vi "Stimulus.Create.vi"(8 "error in (no error)":errorcluster, 11 "State Variables":T1={"NIVS.BaseLogPath"=path "", "NIVS.SystemDefinitionFile"=path "", "NIVS.Events"={"SequenceEvent"=refnum, "SystemChangeEvent"=refnum, "WorkspaceEvent"=refnum}, "NIVS.SequenceState"=enum."Idle", "NIVS.GatewayIPAddress"="", "NIVS.DataLogSpecRef"=refnum, "NIVS.DataLogManagerRef"=refnum, "NIVS.LogSessionGUID"="", "NIVS.WorkspaceManager"=refnum, "NIVS.Deployed"=FALSE, "NIVS.ProfileRef"=refnum, "NIVS.ProfileCallback"=refnum, "NIVS.SystemStateRefs"={"CustDatRef"=refnum, "EvtRef"=refnum, "Target State User Event"=refnum}, "UI.Abort"=refnum, "UI.Pause"=refnum, "UI.EnableLogging"=refnum, "UI.Start"=refnum, "UI.LogChannels"=refnum, "UI.StartIteration"=refnum, "UI.StartStep"=refnum, "UI.Sequence"=refnum, "UI.PreviewMode"=refnum, "UI.Graph"=refnum, "UI.BaseFileName"=refnum, "UI.Profiles"=refnum, "UI.CurrentStep"=refnum, "UI.CurrentIteration"=refnum, "UI.TotalIterations"=refnum, "Sequence.AbortChannel"="", "Sequence.StepInfoChannel"="", "Sequence.Iterations"=0, "Sequence.IterationInfoChannel"="", "Sequence.#ofColumns"=0, "Events.State"=refnum, "Events.Test Result"=refnum, "Events.Progress"=refnum, "INI.Settings"={"Build Location"=path "C:/Simple Sequence Editor/SequenceRepo", "LoggingLocation"=path ""}, "UI.Skip"=refnum, "Sequence.SkipChannel"="", "Restart.Path"=path "", "UI.Duration"=refnum, "Sequence.DurationChannel"=""}) -> (0 "error out":errorcluster, 3 "State Variables":T1={"NIVS.BaseLogPath"=path "", "NIVS.SystemDefinitionFile"=path "", "NIVS.Events"={"SequenceEvent"=refnum, "SystemChangeEvent"=refnum, "WorkspaceEvent"=refnum}, "NIVS.SequenceState"=enum."Idle", "NIVS.GatewayIPAddress"="", "NIVS.DataLogSpecRef"=refnum, "NIVS.DataLogManagerRef"=refnum, "NIVS.LogSessionGUID"="", "NIVS.WorkspaceManager"=refnum, "NIVS.Deployed"=FALSE, "NIVS.ProfileRef"=refnum, "NIVS.ProfileCallback"=refnum, "NIVS.SystemStateRefs"={"CustDatRef"=refnum, "EvtRef"=refnum, "Target State User Event"=refnum}, "UI.Abort"=refnum, "UI.Pause"=refnum, "UI.EnableLogging"=refnum, "UI.Start"=refnum, "UI.LogChannels"=refnum, "UI.StartIteration"=refnum, "UI.StartStep"=refnum, "UI.Sequence"=refnum, "UI.PreviewMode"=refnum, "UI.Graph"=refnum, "UI.BaseFileName"=refnum, "UI.Profiles"=refnum, "UI.CurrentStep"=refnum, "UI.CurrentIteration"=refnum, "UI.TotalIterations"=refnum, "Sequence.AbortChannel"="", "Sequence.StepInfoChannel"="", "Sequence.Iterations"=0, "Sequence.IterationInfoChannel"="", "Sequence.#ofColumns"=0, "Events.State"=refnum, "Events.Test Result"=refnum, "Events.Progress"=refnum, "INI.Settings"={"Build Location"=path "C:/Simple Sequence Editor/SequenceRepo", "LoggingLocation"=path ""}, "UI.Skip"=refnum, "Sequence.SkipChannel"="", "Restart.Path"=path "", "UI.Duration"=refnum, "Sequence.DurationChannel"=""})   [LabVIEW 2015, in "Simple Sequence Tools - Execution.lvlib"]
uses:
  Simple Sequence Tools - Execution.lvlib
  Types/Main.StateVariables.ctl
  Types/Execute.UserEventRefs.ctl
  <vilib>/NI Veristand/Execution/Workspace/SystemStateRegEventRef.ctl
  <vilib>/NI Veristand/Execution/Workspace/Target State Info.ctl
  <vilib>/NI Veristand/Execution/Workspace/Target State.ctl
  Types/Execution.SequenceState.ctl
  <vilib>/NI Veristand/Execution/DataLogging/DataLoggingSpecification Ref.ctl
  NationalInstruments.VeriStand.ClientAPI
  <vilib>/NI Veristand/Execution/DataLogging/IDataLogging Ref.ctl
  <vilib>/NI Veristand/Execution/Workspace/WorkspaceAPI.ctl
  NationalInstruments.VeriStand.RealTimeSequenceDefinitionApi
  <vilib>/NI Veristand/Execution/Workspace/SystemStateEventRef.ctl
  Shared/Types/INI.Settings
  Types/Restart.Settings
  <vilib>/NI Veristand/Execution/DataLogging/TDMS Channel Group.ctl
  <vilib>/NI Veristand/Execution/DataLogging/TDMS Property.ctl
  <vilib>/NI Veristand/Execution/DataLogging/TDMS Channel.ctl
  <vilib>/NI Veristand/Execution/DataLogging/Time Channel Options.ctl
  Types/Log.SelectedChannels.ctl
  NationalInstruments.VeriStand
  NationalInstruments.VeriStand.DataTypes
  <vilib>/NI Veristand/Execution/DataLogging/File Conflict Operation.ctl
  Shared/SubVIs/Main.Constants.vi
  <vilib>/NI Veristand/Execution/DataLogging/New Data Logging Specification (TDMS).vi
  <vilib>/NI Veristand/Execution/DataLogging/Set Data Logging Rate (Target Rate).vi
  <vilib>/NI Veristand/Execution/DataLogging/Set Start Trigger (Start Immediately).vi
  <vilib>/NI Veristand/Execution/Workspace/NI_VS Workspace ExecutionAPI.lvlib
  Shared/Simple Sequence Tools - Shared.lvlib
  <vilib>/NI Veristand/Execution/DataLogging/NI_VS Data Logging API.lvlib
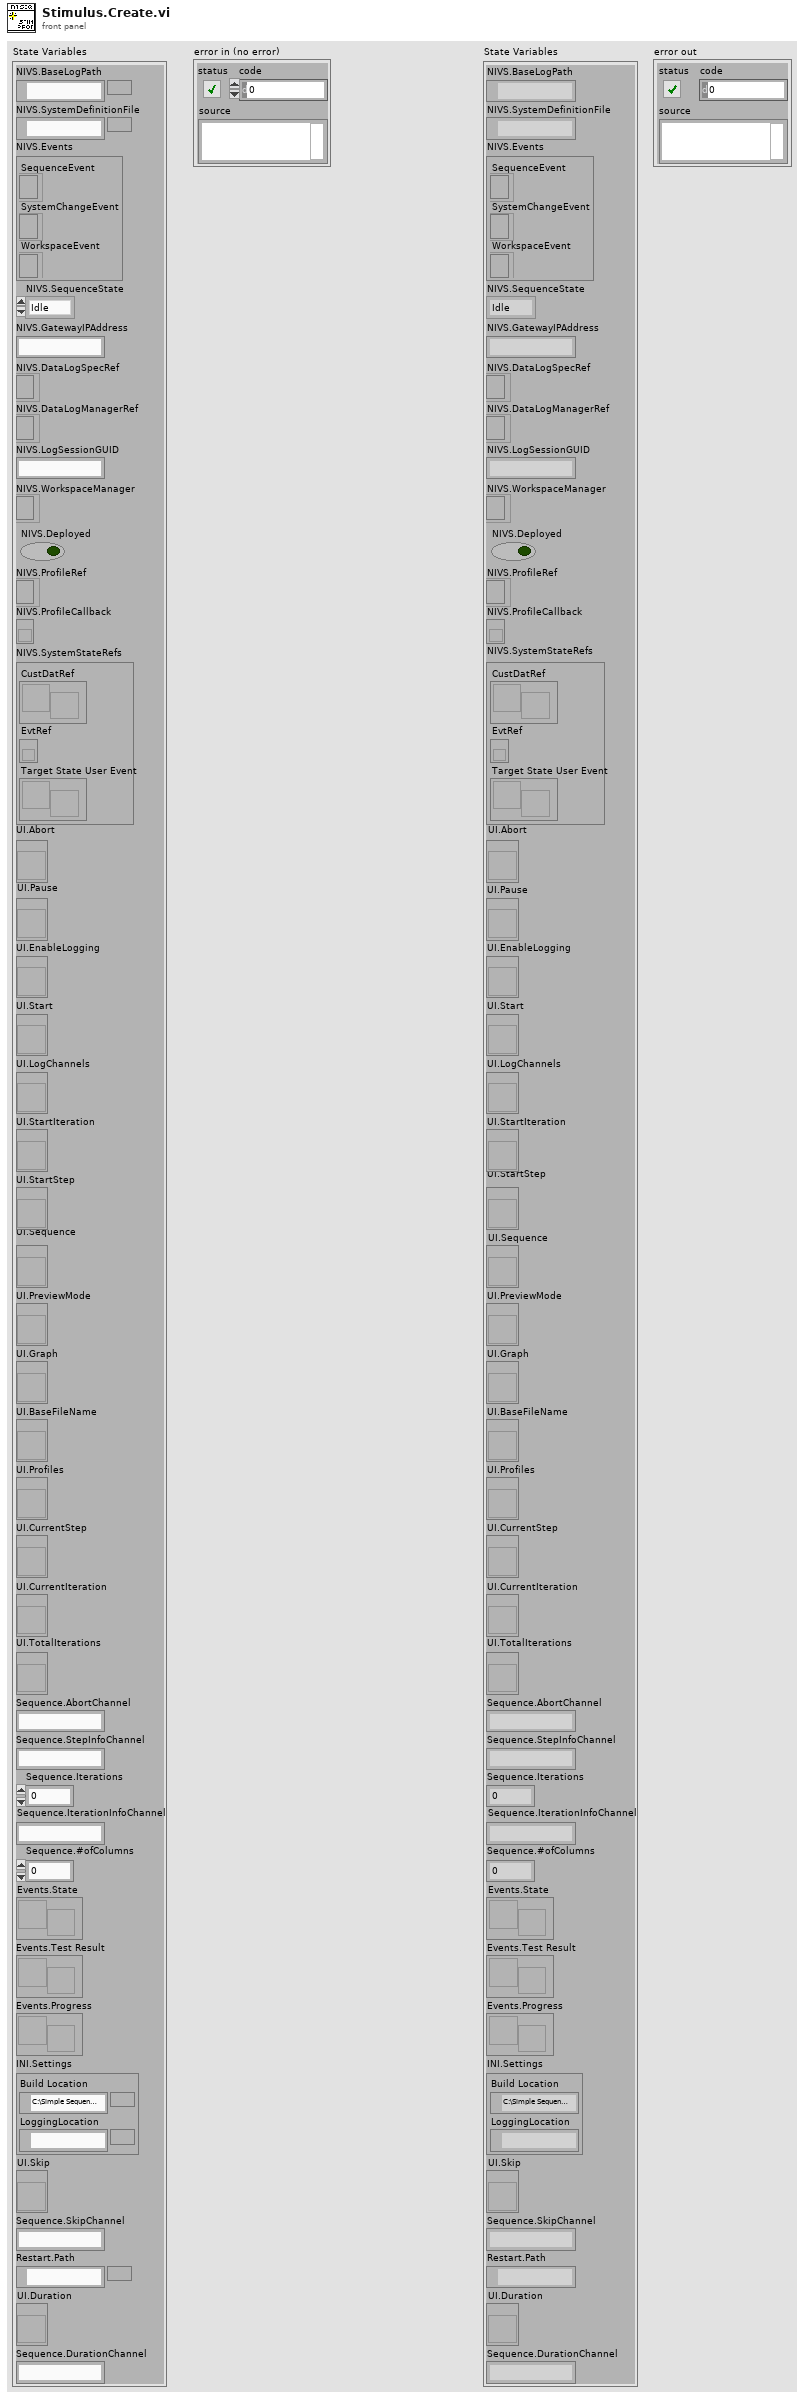
[diagram p1: front panel]
types:
  T1 = typedef "Simple Sequence Tools - Execution.lvlib/Main.StateVariables.ctl" = cluster{"NIVS.BaseLogPath":path, "NIVS.SystemDefinitionFile":path, "NIVS.Events":T2, "NIVS.SequenceState":T4, "NIVS.GatewayIPAddress":string, "NIVS.DataLogSpecRef":T5, "NIVS.DataLogManagerRef":T6, "NIVS.LogSessionGUID":string, "NIVS.WorkspaceManager":T7, "NIVS.Deployed":bool, "NIVS.ProfileRef":refnum<k24>, "NIVS.ProfileCallback":refnum<k27>, "NIVS.SystemStateRefs":T8, "UI.Abort":refnum<vi>, "UI.Pause":refnum<vi>, "UI.EnableLogging":refnum<vi>, "UI.Start":refnum<vi>, "UI.LogChannels":refnum<vi>, "UI.StartIteration":refnum<vi>, "UI.StartStep":refnum<vi>, "UI.Sequence":refnum<vi>, "UI.PreviewMode":refnum<vi>, "UI.Graph":refnum<vi>, "UI.BaseFileName":refnum<vi>, "UI.Profiles":refnum<vi>, "UI.CurrentStep":refnum<vi>, "UI.CurrentIteration":refnum<vi>, "UI.TotalIterations":refnum<vi>, "Sequence.AbortChannel":string, "Sequence.StepInfoChannel":string, "Sequence.Iterations":u32, "Sequence.IterationInfoChannel":string, "Sequence.#ofColumns":i32, "Events.State":refnum<user-event>, "Events.Test Result":refnum<user-event>, "Events.Progress":refnum<user-event>, "INI.Settings":T9, "UI.Skip":refnum<vi>, "Sequence.SkipChannel":string, "Restart.Path":path, "UI.Duration":refnum<vi>, "Sequence.DurationChannel":string}
  T2 = typedef "Simple Sequence Tools - Execution.lvlib/Execute.UserEventRefs.ctl" = cluster{"SequenceEvent":refnum<event-registration>, "SystemChangeEvent":T3, "WorkspaceEvent":refnum<event-registration>}
  T3 = typedef "NI_VS Workspace ExecutionAPI.lvlib/SystemStateRegEventRef.ctl" = refnum<event-registration>
  T4 = typedef "Simple Sequence Tools - Execution.lvlib/Execution.SequenceState.ctl" = enum16{"Idle", "Initializing", "Running", "Paused", "Finalizing", "Complete"}
  T5 = typedef "NI_VS Data Logging API.lvlib/DataLoggingSpecification Ref.ctl" = refnum<k24>
  T6 = typedef "NI_VS Data Logging API.lvlib/IDataLogging Ref.ctl" = refnum<k24>
  T7 = typedef "NI_VS Workspace ExecutionAPI.lvlib/WorkspaceAPI.ctl" = refnum<k24>
  T8 = typedef "NI_VS Workspace ExecutionAPI.lvlib/SystemStateEventRef.ctl" = cluster{"CustDatRef":refnum<user-event>, "EvtRef":refnum<k27>, "Target State User Event":refnum<user-event>}
  T9 = typedef "Simple Sequence Tools - Shared.lvlib/INI.Settings" = cluster{"Build Location":path, "LoggingLocation":path}
  T10 = typedef "Simple Sequence Tools - Execution.lvlib/Restart.Settings" = cluster{"LogFile":path, "Log Settings":T11[], "StimulusProfile":path, "StopIteration":u32, "StopStep":u32, "Log Channels":T15, "Base File Name":string, "Enable Logging":bool, "Profile":string, "StopDuration":dbl}
  T11 = typedef "NI_VS Data Logging API.lvlib/TDMS Channel Group.ctl" = cluster{"Group Name":string, "Group Description":string, "Group Properties":T12[], "Channels":T13[], "Time Channel Options":T14, "Time Channel Name":string}
  T12 = typedef "NI_VS Data Logging API.lvlib/TDMS Property.ctl" = cluster{"Name":string, "Value":variant}
  T13 = typedef "NI_VS Data Logging API.lvlib/TDMS Channel.ctl" = cluster{"Channel Name":string, "Channel Path":string, "Channel Description":string, "Channel Properties":T12[]}
  T14 = typedef "NI_VS Data Logging API.lvlib/Time Channel Options.ctl" = enum16{"No Time Channel", "Absolute Time", "System Time", "System Time - Microseconds", "Absolute Time as Double", "Relative To First Start Trigger", "Relative To Session Start"}
  T15 = typedef "Simple Sequence Tools - Execution.lvlib/Log.SelectedChannels.ctl" = enum16{"Channels (No System Channel)", "Aliases", "All"}
  T16 = enum16{"Channels (No System Channel)", "Aliases", "All"}
  T17 = typedef "NI_VS Data Logging API.lvlib/File Conflict Operation.ctl" = enum16{"Create Unique", "Append to Existing", "Overwrite"}
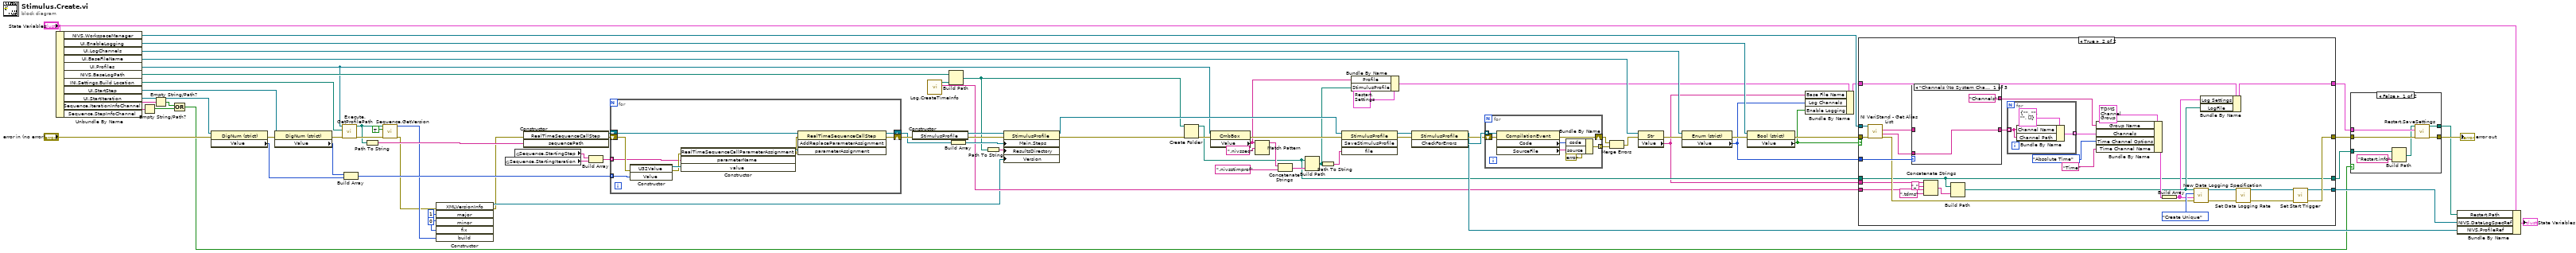
[diagram p0: block diagram]
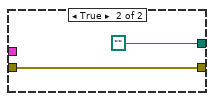
[diagram p2: hidden frame]
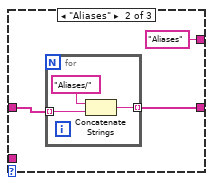
[diagram p4: hidden frame]
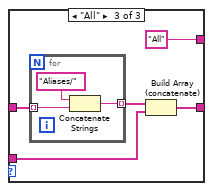
[diagram p5: hidden frame]
diagram:
  w21 = u32 0 ("minor")
  n1 = Unbundle By Name("State Variables") -> ("NIVS.WorkspaceManager"=w51:T7, "UI.EnableLogging"=w53:refnum<vi>, "UI.LogChannels"=w47:refnum<vi>, "UI.BaseFileName"=w48:refnum<vi>, "UI.Profiles"=w33:refnum<vi>, "NIVS.BaseLogPath"=w44:path, "INI.Settings.Build Location"=w1:path, "UI.StartStep"=w61:refnum<vi>, "UI.StartIteration"=w63:refnum<vi>, "Sequence.IterationInfoChannel"=w19:string, "Sequence.StepInfoChannel"=w18:string)
  n2 = Empty String/Path?(string/path=w18) -> (empty?=w16:bool)
  n3 = Empty String/Path?(string/path=w19) -> (empty?=w17:bool)
  n4 = Compound Arithmetic op=OR(w17, w16) -> (w7:bool)
  n5 = property class="DigNum (strict)"(reference=w63, error in="error in (no error)") -> (error out=w62:errorcluster, "Value"=w36:u32)  [unwired: 1 out]
  n6 = property class="DigNum (strict)"(reference=w61, error in=w62) -> (error out=w60:errorcluster, "Value"=w37:u32)  [unwired: 1 out]
  n7 = call "Execute.GetProfilePath.vi"("error in (no error)"=w60, "base path"=w1, "Profiles"=w33) -> ("error out"=w29:errorcluster, "Path"=w28:path)  [unwired: 7 in]
  n8 = Build Array(w37, w36) -> (w59:u32[])
  n9 = Path To String(path=w28) -> (string=w79:string)
  n10 = call "Sequence.GetVersion.vi"("error in (no error)"=w29, "Exists"=TRUE, "Path"=w28) -> ("error out"=w24:errorcluster, "Build"=w25:u32)  [unwired: 7 in]
  n11 = constructor class="XMLVersionInfo"(error in=w24, "major"=u32 1, "minor"=w21, "fix"=w21, "build"=w25) -> (reference out=w26:refnum<k24>, error out=w23:errorcluster)  [unwired: 2 in, 5 out]
  n12 = global read "Main.Constants.vi" "Sequence.StartingIteration"() -> (w57:string)
  n13 = global read "Main.Constants.vi" "Sequence.StartingStep"() -> (w58:string)
  n14 = constructor class="RealTimeSequenceCallStep"(error in=w23, "sequencePath"=w79) -> (reference out=w66:refnum<k24>, error out=w64:errorcluster)  [unwired: 2 in, 2 out]
  n15 = Build Array(w58, w57) -> (w56:string[])
  n16 = for {
    tunnel: w56 -> [w84] mode=indexing
    tunnel: w59 -> [w82] mode=indexing
    shift-right: [w89] -> w65
    shift-left: w66 -> [w90]
    shift-right: [w91] -> w67
    shift-left: w64 -> [w85]
    n17 = constructor class="U32Value"(error in=w85, "Value"=w82) -> (reference out=w87:refnum<k24>, error out=w86:errorcluster)  [unwired: 2 in, 2 out]
    n18 = constructor class="RealTimeSequenceCallParameterAs"(error in=w86, "parameterName"=w84, "value"=w87) -> (reference out=w88:refnum<k24>, error out=w83:errorcluster)  [unwired: 2 in, 3 out]
    n19 = invoke class="RealTimeSequenceCallStep" method="AddReplaceParameterAssignment"(reference=w90, error in=w83, "parameterAssignment"=w88) -> (reference out=w89:refnum<k24>, error out=w91:errorcluster)  [unwired: 1 in, 2 out]
  }
  n20 = constructor class="StimulusProfile"(error in=w67) -> (reference out=w78:refnum<k24>, error out=w75:errorcluster)  [unwired: 2 in, 1 out]
  n21 = call "Log.CreateTimeInfo.vi"() -> ("String"=w40:string, "File Folder"=w43:path)  [unwired: 10 in]
  n22 = Build Path(base path=w44, name or relative path=w43) -> (appended path=w35:path)
  n23 = Build Array(w65) -> (w76:refnum<k24>[])
  n24 = Path To String(path=w35) -> (string=w34:string)
  n25 = property class="StimulusProfile"(reference=w78, error in=w75, "Main.Steps"=w76, "ResultsDirectory"=w34, "Version"=w26) -> (reference out=w55:refnum<k24>, error out=w20:errorcluster)
  n26 = Create Folder(path (use dialog)=w35, error in=w20) -> (created path=w30:path, error out=w32:errorcluster)  [unwired: 1 in, 1 out]
  n27 = property class="CmbBox"(reference=w33, error in=w32) -> (error out=w31:errorcluster, "Value"=w14:string)  [unwired: 1 out]
  n28 = Match Pattern(string=w14, regular expression=".nivsseq" ("string")) -> (before substring=w39:string)  [unwired: 1 in, 3 out]
  n29 = Concatenate Strings(w39, ".nivsstimprof" ("string")) -> (w41:string)
  n30 = Build Path(base path=w30, name or relative path=w41) -> (appended path=w13:path)
  n31 = Path To String(path=w13) -> (string=w77:string)
  n32 = invoke class="StimulusProfile" method="SaveStimulusProfile"(reference=w55, error in=w31, "file"=w77) -> (reference out=w73:refnum<k24>, error out=w72:errorcluster)  [unwired: 1 in, 2 out]
  n33 = Bundle By Name(cluster=T10 {"LogFile"=path "", "Log Settings"=[], "StimulusProfile"=path "", "StopIteration"=0, "StopStep"=0, "Log Channels"=enum."Aliases", "Base File Name"="Log", "Enable Logging"=TRUE, "Profile"="", "StopDuration"=0.0}, "Profile"=w14, "StimulusProfile"=w13) -> (w9:T10)
  n34 = invoke class="StimulusProfile" method="CheckForErrors"(reference=w73, error in=w72) -> (reference out=w45:refnum<k24>, error out=w70:errorcluster, "CheckForErrors"=w71:refnum<k24>[])  [unwired: 1 in]
  n35 = for {
    tunnel: w71 -> [w98] mode=indexing
    tunnel: [w93] -> w68 mode=indexing
    shift-right: [w92] -> w69
    shift-left: w70 -> [w97]
    n36 = property class="CompilationEvent"(reference=w98, error in=w97) -> (error out=w92:errorcluster, "Code"=w95:i32, "SourceFile"=w94:string)  [unwired: 1 out]
    n37 = Bundle By Name(cluster=errorcluster {"status"=TRUE, "code"=0, "source"=""} ("error out"), "code"=w95, "source"=w94) -> (w93:errorcluster)
  }
  n38 = Merge Errors(w69, w68) -> (w46:errorcluster)
  n39 = property class="Str"(reference=w48, error in=w46) -> (error out=w74:errorcluster, "Value"=w12:string)  [unwired: 1 out]
  n40 = property class="Enum (strict)"(reference=w47, error in=w74) -> (error out=w50:errorcluster, "Value"=w11:T16)  [unwired: 1 out]
  n41 = property class="Bool (strict)"(reference=w53, error in=w50) -> (error out=w52:errorcluster, "Value"=w10:bool)  [unwired: 1 out]
  n42 = Bundle By Name(cluster=w9, "Base File Name"=w12, "Log Channels"=w11, "Enable Logging"=w10) -> (w8:T10)
  n43 = case shown="True" w10 {
    tunnel: w52 -> [w101 w131]
    tunnel: [w101 w114] -> w5
    tunnel: w12 -> [_ w104]
    tunnel: w11 -> [_ w129]
    tunnel: w51 -> [_ w130]
    tunnel: [_ w113] -> w54
    tunnel: w30 -> [w99 w102]
    tunnel: w40 -> [_ w108]
    tunnel: w8 -> [w100 w107]
    tunnel: [w100 w103] -> w4
    tunnel: [w99 w102] -> w3
    frame False {
    }
    frame True {
      n44 = call <vilib>:"NI VeriStand - Get Alias List.vi"("error in (no error)"=w131, "WorkspaceManager in"=w130) -> ("error out"=w112:errorcluster, "Channels"=w126:string[], "Aliases"=w128:string[])  [unwired: 6 in, 1 out]
      n45 = case shown="\"Channels (No System Channel)\"" w129 {
        tunnel: w128 -> [_ w136 w144]
        tunnel: [w133 w135 w142] -> w127
        tunnel: w126 -> [w133 _ w141]
        tunnel: ["Channels" "Aliases" "All"] -> w119
        frame "Channels (No System Channel)" {
        }
        frame "Aliases" {
          n46 = for {
            tunnel: w136 -> [w139] mode=indexing
            tunnel: [w137] -> w135 mode=indexing
            n47 = Concatenate Strings("Aliases/", w139) -> (w137:string)
          }
        }
        frame "All" {
          n48 = for {
            tunnel: w144 -> [w147] mode=indexing
            tunnel: [w145] -> w143 mode=indexing
            n49 = Concatenate Strings("Aliases/", w147) -> (w145:string)
          }
          n50 = Build Array (concatenate)(w143, w141) -> (w142:string[])
        }
      }
      n51 = Concatenate Strings(w104, "_" ("string"), w108, ".tdms" ("string")) -> (w110:string)
      n52 = Build Path(base path=w102, name or relative path=w110) -> (appended path=w106:path)
      n53 = for {
        tunnel: w127 -> [w149] mode=indexing
        tunnel: [w148] -> w122 mode=indexing
        n54 = Bundle By Name(cluster=T13 {"Channel Name"="", "Channel Path"="", "Channel Description"="", "Channel Properties"=[]} ("TDMS Channel"), "Channel Name"=w149, "Channel Path"=w149) -> (w148:T13)
      }
      n55 = Bundle By Name(cluster=T11 {"Group Name"="", "Group Description"="", "Group Properties"=[], "Channels"=[], "Time Channel Options"=enum."No Time Channel", "Time Channel Name"=""} ("TDMS Channel Group"), "Group Name"=w119, "Channels"=w122, "Time Channel Options"=Time_Channel_Options."Absolute Time", "Time Channel Name"="Time") -> (w116:T11)
      n56 = Build Array(w116) -> (w105:T11[])
      n57 = call-poly <vilib>:"New Data Logging Specification.vi"("error in (no error)"=w112, "Channel Groups"=w105, "File Conflict Operation"=File_Conflict_Operation."Create Unique", "Base Log File Path"=w106) -> ("error out"=w117:errorcluster, "Data Logging Specification Ref out"=w125:T5)  [unwired: 6 in]
      n58 = Bundle By Name(cluster=w107, "Log Settings"=w105, "LogFile"=w106) -> (w103:T10)
      n59 = call-poly <vilib>:"Set Data Logging Rate.vi"("error in (no error)"=w117, "Data Logging Specification Ref in"=w125) -> ("error out"=w118:errorcluster, "Data Logging Specification Ref out"=w124:T5)  [unwired: 8 in]
      n60 = call-poly <vilib>:"Set Start Trigger.vi"("error in (no error)"=w118, "Data Logging Specification Ref in"=w124) -> ("error out"=w114:errorcluster, "Data Logging Specification Ref out"=w113:T5)  [unwired: 8 in]
    }
  }
  n61 = case shown="False" w7 {
    tunnel: [w156 w159] -> w6
    tunnel: w5 -> [w157 w159]
    tunnel: w4 -> [w155 _]
    tunnel: w3 -> [w154 _]
    tunnel: [w151 path ""] -> w2
    frame False {
      n62 = Build Path(base path=w154, name or relative path="Restart.info") -> (appended path=w152:path)
      n63 = call "Restart.SaveSettings.vi"("error in"=w157, "Restart Settings"=w155, "datalog path (use dialog)"=w152) -> ("error out"=w156:errorcluster, "path"=w151:path)  [unwired: 7 in]
    }
    frame True {
    }
  }
  "error out" <- w6
  n64 = Bundle By Name(cluster="State Variables", "Restart.Path"=w2, "NIVS.DataLogSpecRef"=w54, "NIVS.ProfileRef"=w45) -> (→"State Variables":T1)
